vi "App - analyze RUS V6.vi"() -> ()   [LabVIEW 2018] (continued)
"timestamp"=timestamp(3493798379 s since 1904-01-01), "Magn Field(T)"=0.0}, {"temperature"=62.245, "lorentzian"={"A (VHz)"=0.0, "f (Hz)"=0.0, "G (Hz)"=0.0, "phi(rad)"=0.0, "Q"=0.0, "Norm  Ampl"=0.0, "bg (V)"=0.0+0.0i, "4corners"={"z (-pi/2)"=0.0+0.0i, "z(inf)"=0.0+0.0i, "z (pi/2)"=0.0+0.0i, "z center"=0.0+0.0i, "z(0)"=0.0+0.0i, "radius"=0.0}}, "timestamp(min)"=1177.3000000044703, "timestamp"=timestamp(3493798459 s since 1904-01-01), "Magn Field(T)"=0.0}, {"temperature"=62.184, "lorentzian"={"A (VHz)"=0.0, "f (Hz)"=0.0, "G (Hz)"=0.0, "phi(rad)"=0.0, "Q"=0.0, "Norm  Ampl"=0.0, "bg (V)"=0.0+0.0i, "4corners"={"z (-pi/2)"=0.0+0.0i, "z(inf)"=0.0+0.0i, "z (pi/2)"=0.0+0.0i, "z center"=0.0+0.0i, "z(0)"=0.0+0.0i, "radius"=0.0}}, "timestamp(min)"=1178.6166666671634, "timestamp"=timestamp(3493798538 s since 1904-01-01), "Magn Field(T)"=0.0}, {"temperature"=62.127, "lorentzian"={"A (VHz)"=0.0, "f (Hz)"=0.0, "G (Hz)"=0.0, "phi(rad)"=0.0, "Q"=0.0, "Norm  Ampl"=0.0, "bg (V)"=0.0+0.0i, "4corners"={"z (-pi/2)"=0.0+0.0i, "z(inf)"=0.0+0.0i, "z (pi/2)"=0.0+0.0i, "z center"=0.0+0.0i, "z(0)"=0.0+0.0i, "radius"=0.0}}, "timestamp(min)"=1179.933333337307, "timestamp"=timestamp(3493798617 s since 1904-01-01), "Magn Field(T)"=0.0}, {"temperature"=62.069, "lorentzian"={"A (VHz)"=0.0, "f (Hz)"=0.0, "G (Hz)"=0.0, "phi(rad)"=0.0, "Q"=0.0, "Norm  Ampl"=0.0, "bg (V)"=0.0+0.0i, "4corners"={"z (-pi/2)"=0.0+0.0i, "z(inf)"=0.0+0.0i, "z (pi/2)"=0.0+0.0i, "z center"=0.0+0.0i, "z(0)"=0.0+0.0i, "radius"=0.0}}, "timestamp(min)"=1181.2666666656733, "timestamp"=timestamp(3493798697 s since 1904-01-01), "Magn Field(T)"=0.0}, {"temperature"=62.01, "lorentzian"={"A (VHz)"=0.0, "f (Hz)"=0.0, "G (Hz)"=0.0, "phi(rad)"=0.0, "Q"=0.0, "Norm  Ampl"=0.0, "bg (V)"=0.0+0.0i, "4corners"={"z (-pi/2)"=0.0+0.0i, "z(inf)"=0.0+0.0i, "z (pi/2)"=0.0+0.0i, "z center"=0.0+0.0i, "z(0)"=0.0+0.0i, "radius"=0.0}}, "timestamp(min)"=1182.5833333358169, "timestamp"=timestamp(3493798776 s since 1904-01-01), "Magn Field(T)"=0.0}, {"temperature"=61.951, "lorentzian"={"A (VHz)"=0.0, "f (Hz)"=0.0, "G (Hz)"=0.0, "phi(rad)"=0.0, "Q"=0.0, "Norm  Ampl"=0.0, "bg (V)"=0.0+0.0i, "4corners"={"z (-pi/2)"=0.0+0.0i, "z(inf)"=0.0+0.0i, "z (pi/2)"=0.0+0.0i, "z center"=0.0+0.0i, "z(0)"=0.0+0.0i, "radius"=0.0}}, "timestamp(min)"=1183.8999999985099, "timestamp"=timestamp(3493798855 s since 1904-01-01), "Magn Field(T)"=0.0}, {"temperature"=61.895, "lorentzian"={"A (VHz)"=0.0, "f (Hz)"=0.0, "G (Hz)"=0.0, "phi(rad)"=0.0, "Q"=0.0, "Norm  Ampl"=0.0, "bg (V)"=0.0+0.0i, "4corners"={"z (-pi/2)"=0.0+0.0i, "z(inf)"=0.0+0.0i, "z (pi/2)"=0.0+0.0i, "z center"=0.0+0.0i, "z(0)"=0.0+0.0i, "radius"=0.0}}, "timestamp(min)"=1185.2333333343267, "timestamp"=timestamp(3493798935 s since 1904-01-01), "Magn Field(T)"=0.0}, {"temperature"=61.834, "lorentzian"={"A (VHz)"=0.0, "f (Hz)"=0.0, "G (Hz)"=0.0, "phi(rad)"=0.0, "Q"=0.0, "Norm  Ampl"=0.0, "bg (V)"=0.0+0.0i, "4corners"={"z (-pi/2)"=0.0+0.0i, "z(inf)"=0.0+0.0i, "z (pi/2)"=0.0+0.0i, "z center"=0.0+0.0i, "z(0)"=0.0+0.0i, "radius"=0.0}}, "timestamp(min)"=1186.5500000044703, "timestamp"=timestamp(3493799014 s since 1904-01-01), "Magn Field(T)"=0.0}, {"temperature"=61.775, "lorentzian"={"A (VHz)"=0.0, "f (Hz)"=0.0, "G (Hz)"=0.0, "phi(rad)"=0.0, "Q"=0.0, "Norm  Ampl"=0.0, "bg (V)"=0.0+0.0i, "4corners"={"z (-pi/2)"=0.0+0.0i, "z(inf)"=0.0+0.0i, "z (pi/2)"=0.0+0.0i, "z center"=0.0+0.0i, "z(0)"=0.0+0.0i, "radius"=0.0}}, "timestamp(min)"=1187.8833333328366, "timestamp"=timestamp(3493799094 s since 1904-01-01), "Magn Field(T)"=0.0}, {"temperature"=61.716, "lorentzian"={"A (VHz)"=0.0, "f (Hz)"=0.0, "G (Hz)"=0.0, "phi(rad)"=0.0, "Q"=0.0, "Norm  Ampl"=0.0, "bg (V)"=0.0+0.0i, "4corners"={"z (-pi/2)"=0.0+0.0i, "z(inf)"=0.0+0.0i, "z (pi/2)"=0.0+0.0i, "z center"=0.0+0.0i, "z(0)"=0.0+0.0i, "radius"=0.0}}, "timestamp(min)"=1189.2000000029802, "timestamp"=timestamp(3493799173 s since 1904-01-01), "Magn Field(T)"=0.0}, {"temperature"=61.656, "lorentzian"={"A (VHz)"=0.0, "f (Hz)"=0.0, "G (Hz)"=0.0, "phi(rad)"=0.0, "Q"=0.0, "Norm  Ampl"=0.0, "bg (V)"=0.0+0.0i, "4corners"={"z (-pi/2)"=0.0+0.0i, "z(inf)"=0.0+0.0i, "z (pi/2)"=0.0+0.0i, "z center"=0.0+0.0i, "z(0)"=0.0+0.0i, "radius"=0.0}}, "timestamp(min)"=1190.5166666656733, "timestamp"=timestamp(3493799252 s since 1904-01-01), "Magn Field(T)"=0.0}, {"temperature"=61.601, "lorentzian"={"A (VHz)"=0.0, "f (Hz)"=0.0, "G (Hz)"=0.0, "phi(rad)"=0.0, "Q"=0.0, "Norm  Ampl"=0.0, "bg (V)"=0.0+0.0i, "4corners"={"z (-pi/2)"=0.0+0.0i, "z(inf)"=0.0+0.0i, "z (pi/2)"=0.0+0.0i, "z center"=0.0+0.0i, "z(0)"=0.0+0.0i, "radius"=0.0}}, "timestamp(min)"=1191.8500000014901, "timestamp"=timestamp(3493799332 s since 1904-01-01), "Magn Field(T)"=0.0}, {"temperature"=61.541, "lorentzian"={"A (VHz)"=0.0, "f (Hz)"=0.0, "G (Hz)"=0.0, "phi(rad)"=0.0, "Q"=0.0, "Norm  Ampl"=0.0, "bg (V)"=0.0+0.0i, "4corners"={"z (-pi/2)"=0.0+0.0i, "z(inf)"=0.0+0.0i, "z (pi/2)"=0.0+0.0i, "z center"=0.0+0.0i, "z(0)"=0.0+0.0i, "radius"=0.0}}, "timestamp(min)"=1193.1666666641831, "timestamp"=timestamp(3493799411 s since 1904-01-01), "Magn Field(T)"=0.0}, {"temperature"=61.482, "lorentzian"={"A (VHz)"=0.0, "f (Hz)"=0.0, "G (Hz)"=0.0, "phi(rad)"=0.0, "Q"=0.0, "Norm  Ampl"=0.0, "bg (V)"=0.0+0.0i, "4corners"={"z (-pi/2)"=0.0+0.0i, "z(inf)"=0.0+0.0i, "z (pi/2)"=0.0+0.0i, "z center"=0.0+0.0i, "z(0)"=0.0+0.0i, "radius"=0.0}}, "timestamp(min)"=1194.5, "timestamp"=timestamp(3493799491 s since 1904-01-01), "Magn Field(T)"=0.0}, {"temperature"=61.424, "lorentzian"={"A (VHz)"=0.0, "f (Hz)"=0.0, "G (Hz)"=0.0, "phi(rad)"=0.0, "Q"=0.0, "Norm  Ampl"=0.0, "bg (V)"=0.0+0.0i, "4corners"={"z (-pi/2)"=0.0+0.0i, "z(inf)"=0.0+0.0i, "z (pi/2)"=0.0+0.0i, "z center"=0.0+0.0i, "z(0)"=0.0+0.0i, "radius"=0.0}}, "timestamp(min)"=1195.8166666701436, "timestamp"=timestamp(3493799570 s since 1904-01-01), "Magn Field(T)"=0.0}, {"temperature"=61.367, "lorentzian"={"A (VHz)"=0.0, "f (Hz)"=0.0, "G (Hz)"=0.0, "phi(rad)"=0.0, "Q"=0.0, "Norm  Ampl"=0.0, "bg (V)"=0.0+0.0i, "4corners"={"z (-pi/2)"=0.0+0.0i, "z(inf)"=0.0+0.0i, "z (pi/2)"=0.0+0.0i, "z center"=0.0+0.0i, "z(0)"=0.0+0.0i, "radius"=0.0}}, "timestamp(min)"=1197.1333333328366, "timestamp"=timestamp(3493799649 s since 1904-01-01), "Magn Field(T)"=0.0}, {"temperature"=61.307, "lorentzian"={"A (VHz)"=0.0, "f (Hz)"=0.0, "G (Hz)"=0.0, "phi(rad)"=0.0, "Q"=0.0, "Norm  Ampl"=0.0, "bg (V)"=0.0+0.0i, "4corners"={"z (-pi/2)"=0.0+0.0i, "z(inf)"=0.0+0.0i, "z (pi/2)"=0.0+0.0i, "z center"=0.0+0.0i, "z(0)"=0.0+0.0i, "radius"=0.0}}, "timestamp(min)"=1198.4666666686535, "timestamp"=timestamp(3493799729 s since 1904-01-01), "Magn Field(T)"=0.0}, {"temperature"=61.247, "lorentzian"={"A (VHz)"=0.0, "f (Hz)"=0.0, "G (Hz)"=0.0, "phi(rad)"=0.0, "Q"=0.0, "Norm  Ampl"=0.0, "bg (V)"=0.0+0.0i, "4corners"={"z (-pi/2)"=0.0+0.0i, "z(inf)"=0.0+0.0i, "z (pi/2)"=0.0+0.0i, "z center"=0.0+0.0i, "z(0)"=0.0+0.0i, "radius"=0.0}}, "timestamp(min)"=1199.7833333313465, "timestamp"=timestamp(3493799808 s since 1904-01-01), "Magn Field(T)"=0.0}, {"temperature"=61.191, "lorentzian"={"A (VHz)"=0.0, "f (Hz)"=0.0, "G (Hz)"=0.0, "phi(rad)"=0.0, "Q"=0.0, "Norm  Ampl"=0.0, "bg (V)"=0.0+0.0i, "4corners"={"z (-pi/2)"=0.0+0.0i, "z(inf)"=0.0+0.0i, "z (pi/2)"=0.0+0.0i, "z center"=0.0+0.0i, "z(0)"=0.0+0.0i, "radius"=0.0}}, "timestamp(min)"=1201.1000000014901, "timestamp"=timestamp(3493799887 s since 1904-01-01), "Magn Field(T)"=0.0}, {"temperature"=61.13, "lorentzian"={"A (VHz)"=0.0, "f (Hz)"=0.0, "G (Hz)"=0.0, "phi(rad)"=0.0, "Q"=0.0, "Norm  Ampl"=0.0, "bg (V)"=0.0+0.0i, "4corners"={"z (-pi/2)"=0.0+0.0i, "z(inf)"=0.0+0.0i, "z (pi/2)"=0.0+0.0i, "z center"=0.0+0.0i, "z(0)"=0.0+0.0i, "radius"=0.0}}, "timestamp(min)"=1202.433333337307, "timestamp"=timestamp(3493799967 s since 1904-01-01), "Magn Field(T)"=0.0}, {"temperature"=61.073, "lorentzian"={"A (VHz)"=0.0, "f (Hz)"=0.0, "G (Hz)"=0.0, "phi(rad)"=0.0, "Q"=0.0, "Norm  Ampl"=0.0, "bg (V)"=0.0+0.0i, "4corners"={"z (-pi/2)"=0.0+0.0i, "z(inf)"=0.0+0.0i, "z (pi/2)"=0.0+0.0i, "z center"=0.0+0.0i, "z(0)"=0.0+0.0i, "radius"=0.0}}, "timestamp(min)"=1203.75, "timestamp"=timestamp(3493800046 s since 1904-01-01), "Magn Field(T)"=0.0}, {"temperature"=61.013, "lorentzian"={"A (VHz)"=0.0, "f (Hz)"=0.0, "G (Hz)"=0.0, "phi(rad)"=0.0, "Q"=0.0, "Norm  Ampl"=0.0, "bg (V)"=0.0+0.0i, "4corners"={"z (-pi/2)"=0.0+0.0i, "z(inf)"=0.0+0.0i, "z (pi/2)"=0.0+0.0i, "z center"=0.0+0.0i, "z(0)"=0.0+0.0i, "radius"=0.0}}, "timestamp(min)"=1205.0833333358169, "timestamp"=timestamp(3493800126 s since 1904-01-01), "Magn Field(T)"=0.0}, {"temperature"=60.953, "lorentzian"={"A (VHz)"=0.0, "f (Hz)"=0.0, "G (Hz)"=0.0, "phi(rad)"=0.0, "Q"=0.0, "Norm  Ampl"=0.0, "bg (V)"=0.0+0.0i, "4corners"={"z (-pi/2)"=0.0+0.0i, "z(inf)"=0.0+0.0i, "z (pi/2)"=0.0+0.0i, "z center"=0.0+0.0i, "z(0)"=0.0+0.0i, "radius"=0.0}}, "timestamp(min)"=1206.3999999985099, "timestamp"=timestamp(3493800205 s since 1904-01-01), "Magn Field(T)"=0.0}, {"temperature"=60.896, "lorentzian"={"A (VHz)"=0.0, "f (Hz)"=0.0, "G (Hz)"=0.0, "phi(rad)"=0.0, "Q"=0.0, "Norm  Ampl"=0.0, "bg (V)"=0.0+0.0i, "4corners"={"z (-pi/2)"=0.0+0.0i, "z(inf)"=0.0+0.0i, "z (pi/2)"=0.0+0.0i, "z center"=0.0+0.0i, "z(0)"=0.0+0.0i, "radius"=0.0}}, "timestamp(min)"=1207.7166666686535, "timestamp"=timestamp(3493800284 s since 1904-01-01), "Magn Field(T)"=0.0}, {"temperature"=60.837, "lorentzian"={"A (VHz)"=0.0, "f (Hz)"=0.0, "G (Hz)"=0.0, "phi(rad)"=0.0, "Q"=0.0, "Norm  Ampl"=0.0, "bg (V)"=0.0+0.0i, "4corners"={"z (-pi/2)"=0.0+0.0i, "z(inf)"=0.0+0.0i, "z (pi/2)"=0.0+0.0i, "z center"=0.0+0.0i, "z(0)"=0.0+0.0i, "radius"=0.0}}, "timestamp(min)"=1209.0500000044703, "timestamp"=timestamp(3493800364 s since 1904-01-01), "Magn Field(T)"=0.0}, {"temperature"=60.781, "lorentzian"={"A (VHz)"=0.0, "f (Hz)"=0.0, "G (Hz)"=0.0, "phi(rad)"=0.0, "Q"=0.0, "Norm  Ampl"=0.0, "bg (V)"=0.0+0.0i, "4corners"={"z (-pi/2)"=0.0+0.0i, "z(inf)"=0.0+0.0i, "z (pi/2)"=0.0+0.0i, "z center"=0.0+0.0i, "z(0)"=0.0+0.0i, "radius"=0.0}}, "timestamp(min)"=1210.3666666671634, "timestamp"=timestamp(3493800443 s since 1904-01-01), "Magn Field(T)"=0.0}, {"temperature"=60.72, "lorentzian"={"A (VHz)"=0.0, "f (Hz)"=0.0, "G (Hz)"=0.0, "phi(rad)"=0.0, "Q"=0.0, "Norm  Ampl"=0.0, "bg (V)"=0.0+0.0i, "4corners"={"z (-pi/2)"=0.0+0.0i, "z(inf)"=0.0+0.0i, "z (pi/2)"=0.0+0.0i, "z center"=0.0+0.0i, "z(0)"=0.0+0.0i, "radius"=0.0}}, "timestamp(min)"=1211.683333337307, "timestamp"=timestamp(3493800522 s since 1904-01-01), "Magn Field(T)"=0.0}, {"temperature"=60.659, "lorentzian"={"A (VHz)"=0.0, "f (Hz)"=0.0, "G (Hz)"=0.0, "phi(rad)"=0.0, "Q"=0.0, "Norm  Ampl"=0.0, "bg (V)"=0.0+0.0i, "4corners"={"z (-pi/2)"=0.0+0.0i, "z(inf)"=0.0+0.0i, "z (pi/2)"=0.0+0.0i, "z center"=0.0+0.0i, "z(0)"=0.0+0.0i, "radius"=0.0}}, "timestamp(min)"=1213.0166666656733, "timestamp"=timestamp(3493800602 s since 1904-01-01), "Magn Field(T)"=0.0}, {"temperature"=60.601, "lorentzian"={"A (VHz)"=0.0, "f (Hz)"=0.0, "G (Hz)"=0.0, "phi(rad)"=0.0, "Q"=0.0, "Norm  Ampl"=0.0, "bg (V)"=0.0+0.0i, "4corners"={"z (-pi/2)"=0.0+0.0i, "z(inf)"=0.0+0.0i, "z (pi/2)"=0.0+0.0i, "z center"=0.0+0.0i, "z(0)"=0.0+0.0i, "radius"=0.0}}, "timestamp(min)"=1214.3333333358169, "timestamp"=timestamp(3493800681 s since 1904-01-01), "Magn Field(T)"=0.0}, {"temperature"=60.545, "lorentzian"={"A (VHz)"=0.0, "f (Hz)"=0.0, "G (Hz)"=0.0, "phi(rad)"=0.0, "Q"=0.0, "Norm  Ampl"=0.0, "bg (V)"=0.0+0.0i, "4corners"={"z (-pi/2)"=0.0+0.0i, "z(inf)"=0.0+0.0i, "z (pi/2)"=0.0+0.0i, "z center"=0.0+0.0i, "z(0)"=0.0+0.0i, "radius"=0.0}}, "timestamp(min)"=1215.6666666641831, "timestamp"=timestamp(3493800761 s since 1904-01-01), "Magn Field(T)"=0.0}, {"temperature"=60.486, "lorentzian"={"A (VHz)"=0.0, "f (Hz)"=0.0, "G (Hz)"=0.0, "phi(rad)"=0.0, "Q"=0.0, "Norm  Ampl"=0.0, "bg (V)"=0.0+0.0i, "4corners"={"z (-pi/2)"=0.0+0.0i, "z(inf)"=0.0+0.0i, "z (pi/2)"=0.0+0.0i, "z center"=0.0+0.0i, "z(0)"=0.0+0.0i, "radius"=0.0}}, "timestamp(min)"=1216.9833333343267, "timestamp"=timestamp(3493800840 s since 1904-01-01), "Magn Field(T)"=0.0}, {"temperature"=60.426, "lorentzian"={"A (VHz)"=0.0, "f (Hz)"=0.0, "G (Hz)"=0.0, "phi(rad)"=0.0, "Q"=0.0, "Norm  Ampl"=0.0, "bg (V)"=0.0+0.0i, "4corners"={"z (-pi/2)"=0.0+0.0i, "z(inf)"=0.0+0.0i, "z (pi/2)"=0.0+0.0i, "z center"=0.0+0.0i, "z(0)"=0.0+0.0i, "radius"=0.0}}, "timestamp(min)"=1218.3000000044703, "timestamp"=timestamp(3493800919 s since 1904-01-01), "Magn Field(T)"=0.0}, {"temperature"=60.367, "lorentzian"={"A (VHz)"=0.0, "f (Hz)"=0.0, "G (Hz)"=0.0, "phi(rad)"=0.0, "Q"=0.0, "Norm  Ampl"=0.0, "bg (V)"=0.0+0.0i, "4corners"={"z (-pi/2)"=0.0+0.0i, "z(inf)"=0.0+0.0i, "z (pi/2)"=0.0+0.0i, "z center"=0.0+0.0i, "z(0)"=0.0+0.0i, "radius"=0.0}}, "timestamp(min)"=1219.6333333328366, "timestamp"=timestamp(3493800999 s since 1904-01-01), "Magn Field(T)"=0.0}, {"temperature"=60.308, "lorentzian"={"A (VHz)"=0.0, "f (Hz)"=0.0, "G (Hz)"=0.0, "phi(rad)"=0.0, "Q"=0.0, "Norm  Ampl"=0.0, "bg (V)"=0.0+0.0i, "4corners"={"z (-pi/2)"=0.0+0.0i, "z(inf)"=0.0+0.0i, "z (pi/2)"=0.0+0.0i, "z center"=0.0+0.0i, "z(0)"=0.0+0.0i, "radius"=0.0}}, "timestamp(min)"=1220.9500000029802, "timestamp"=timestamp(3493801078 s since 1904-01-01), "Magn Field(T)"=0.0}, {"temperature"=60.248, "lorentzian"={"A (VHz)"=0.0, "f (Hz)"=0.0, "G (Hz)"=0.0, "phi(rad)"=0.0, "Q"=0.0, "Norm  Ampl"=0.0, "bg (V)"=0.0+0.0i, "4corners"={"z (-pi/2)"=0.0+0.0i, "z(inf)"=0.0+0.0i, "z (pi/2)"=0.0+0.0i, "z center"=0.0+0.0i, "z(0)"=0.0+0.0i, "radius"=0.0}}, "timestamp(min)"=1222.2833333313465, "timestamp"=timestamp(3493801158 s since 1904-01-01), "Magn Field(T)"=0.0}, {"temperature"=60.19, "lorentzian"={"A (VHz)"=0.0, "f (Hz)"=0.0, "G (Hz)"=0.0, "phi(rad)"=0.0, "Q"=0.0, "Norm  Ampl"=0.0, "bg (V)"=0.0+0.0i, "4corners"={"z (-pi/2)"=0.0+0.0i, "z(inf)"=0.0+0.0i, "z (pi/2)"=0.0+0.0i, "z center"=0.0+0.0i, "z(0)"=0.0+0.0i, "radius"=0.0}}, "timestamp(min)"=1223.6000000014901, "timestamp"=timestamp(3493801237 s since 1904-01-01), "Magn Field(T)"=0.0}, {"temperature"=60.133, "lorentzian"={"A (VHz)"=0.0, "f (Hz)"=0.0, "G (Hz)"=0.0, "phi(rad)"=0.0, "Q"=0.0, "Norm  Ampl"=0.0, "bg (V)"=0.0+0.0i, "4corners"={"z (-pi/2)"=0.0+0.0i, "z(inf)"=0.0+0.0i, "z (pi/2)"=0.0+0.0i, "z center"=0.0+0.0i, "z(0)"=0.0+0.0i, "radius"=0.0}}, "timestamp(min)"=1224.9166666641831, "timestamp"=timestamp(3493801316 s since 1904-01-01), "Magn Field(T)"=0.0}, {"temperature"=60.073, "lorentzian"={"A (VHz)"=0.0, "f (Hz)"=0.0, "G (Hz)"=0.0, "phi(rad)"=0.0, "Q"=0.0, "Norm  Ampl"=0.0, "bg (V)"=0.0+0.0i, "4corners"={"z (-pi/2)"=0.0+0.0i, "z(inf)"=0.0+0.0i, "z (pi/2)"=0.0+0.0i, "z center"=0.0+0.0i, "z(0)"=0.0+0.0i, "radius"=0.0}}, "timestamp(min)"=1226.25, "timestamp"=timestamp(3493801396 s since 1904-01-01), "Magn Field(T)"=0.0}, {"temperature"=60.013, "lorentzian"={"A (VHz)"=0.0, "f (Hz)"=0.0, "G (Hz)"=0.0, "phi(rad)"=0.0, "Q"=0.0, "Norm  Ampl"=0.0, "bg (V)"=0.0+0.0i, "4corners"={"z (-pi/2)"=0.0+0.0i, "z(inf)"=0.0+0.0i, "z (pi/2)"=0.0+0.0i, "z center"=0.0+0.0i, "z(0)"=0.0+0.0i, "radius"=0.0}}, "timestamp(min)"=1227.5666666701436, "timestamp"=timestamp(3493801475 s since 1904-01-01), "Magn Field(T)"=0.0}, {"temperature"=59.955, "lorentzian"={"A (VHz)"=0.0, "f (Hz)"=0.0, "G (Hz)"=0.0, "phi(rad)"=0.0, "Q"=0.0, "Norm  Ampl"=0.0, "bg (V)"=0.0+0.0i, "4corners"={"z (-pi/2)"=0.0+0.0i, "z(inf)"=0.0+0.0i, "z (pi/2)"=0.0+0.0i, "z center"=0.0+0.0i, "z(0)"=0.0+0.0i, "radius"=0.0}}, "timestamp(min)"=1228.8833333328366, "timestamp"=timestamp(3493801554 s since 1904-01-01), "Magn Field(T)"=0.0}, {"temperature"=59.894, "lorentzian"={"A (VHz)"=0.0, "f (Hz)"=0.0, "G (Hz)"=0.0, "phi(rad)"=0.0, "Q"=0.0, "Norm  Ampl"=0.0, "bg (V)"=0.0+0.0i, "4corners"={"z (-pi/2)"=0.0+0.0i, "z(inf)"=0.0+0.0i, "z (pi/2)"=0.0+0.0i, "z center"=0.0+0.0i, "z(0)"=0.0+0.0i, "radius"=0.0}}, "timestamp(min)"=1230.2166666686535, "timestamp"=timestamp(3493801634 s since 1904-01-01), "Magn Field(T)"=0.0}, {"temperature"=59.839, "lorentzian"={"A (VHz)"=0.0, "f (Hz)"=0.0, "G (Hz)"=0.0, "phi(rad)"=0.0, "Q"=0.0, "Norm  Ampl"=0.0, "bg (V)"=0.0+0.0i, "4corners"={"z (-pi/2)"=0.0+0.0i, "z(inf)"=0.0+0.0i, "z (pi/2)"=0.0+0.0i, "z center"=0.0+0.0i, "z(0)"=0.0+0.0i, "radius"=0.0}}, "timestamp(min)"=1231.5333333313465, "timestamp"=timestamp(3493801713 s since 1904-01-01), "Magn Field(T)"=0.0}, {"temperature"=59.776, "lorentzian"={"A (VHz)"=0.0, "f (Hz)"=0.0, "G (Hz)"=0.0, "phi(rad)"=0.0, "Q"=0.0, "Norm  Ampl"=0.0, "bg (V)"=0.0+0.0i, "4corners"={"z (-pi/2)"=0.0+0.0i, "z(inf)"=0.0+0.0i, "z (pi/2)"=0.0+0.0i, "z center"=0.0+0.0i, "z(0)"=0.0+0.0i, "radius"=0.0}}, "timestamp(min)"=1232.8666666671634, "timestamp"=timestamp(3493801793 s since 1904-01-01), "Magn Field(T)"=0.0}, {"temperature"=59.72, "lorentzian"={"A (VHz)"=0.0, "f (Hz)"=0.0, "G (Hz)"=0.0, "phi(rad)"=0.0, "Q"=0.0, "Norm  Ampl"=0.0, "bg (V)"=0.0+0.0i, "4corners"={"z (-pi/2)"=0.0+0.0i, "z(inf)"=0.0+0.0i, "z (pi/2)"=0.0+0.0i, "z center"=0.0+0.0i, "z(0)"=0.0+0.0i, "radius"=0.0}}, "timestamp(min)"=1234.183333337307, "timestamp"=timestamp(3493801872 s since 1904-01-01), "Magn Field(T)"=0.0}, {"temperature"=59.661, "lorentzian"={"A (VHz)"=0.0, "f (Hz)"=0.0, "G (Hz)"=0.0, "phi(rad)"=0.0, "Q"=0.0, "Norm  Ampl"=0.0, "bg (V)"=0.0+0.0i, "4corners"={"z (-pi/2)"=0.0+0.0i, "z(inf)"=0.0+0.0i, "z (pi/2)"=0.0+0.0i, "z center"=0.0+0.0i, "z(0)"=0.0+0.0i, "radius"=0.0}}, "timestamp(min)"=1235.5, "timestamp"=timestamp(3493801951 s since 1904-01-01), "Magn Field(T)"=0.0}, {"temperature"=59.598, "lorentzian"={"A (VHz)"=0.0, "f (Hz)"=0.0, "G (Hz)"=0.0, "phi(rad)"=0.0, "Q"=0.0, "Norm  Ampl"=0.0, "bg (V)"=0.0+0.0i, "4corners"={"z (-pi/2)"=0.0+0.0i, "z(inf)"=0.0+0.0i, "z (pi/2)"=0.0+0.0i, "z center"=0.0+0.0i, "z(0)"=0.0+0.0i, "radius"=0.0}}, "timestamp(min)"=1236.8333333358169, "timestamp"=timestamp(3493802031 s since 1904-01-01), "Magn Field(T)"=0.0}, {"temperature"=59.54, "lorentzian"={"A (VHz)"=0.0, "f (Hz)"=0.0, "G (Hz)"=0.0, "phi(rad)"=0.0, "Q"=0.0, "Norm  Ampl"=0.0, "bg (V)"=0.0+0.0i, "4corners"={"z (-pi/2)"=0.0+0.0i, "z(inf)"=0.0+0.0i, "z (pi/2)"=0.0+0.0i, "z center"=0.0+0.0i, "z(0)"=0.0+0.0i, "radius"=0.0}}, "timestamp(min)"=1238.1499999985099, "timestamp"=timestamp(3493802110 s since 1904-01-01), "Magn Field(T)"=0.0}, {"temperature"=59.481, "lorentzian"={"A (VHz)"=0.0, "f (Hz)"=0.0, "G (Hz)"=0.0, "phi(rad)"=0.0, "Q"=0.0, "Norm  Ampl"=0.0, "bg (V)"=0.0+0.0i, "4corners"={"z (-pi/2)"=0.0+0.0i, "z(inf)"=0.0+0.0i, "z (pi/2)"=0.0+0.0i, "z center"=0.0+0.0i, "z(0)"=0.0+0.0i, "radius"=0.0}}, "timestamp(min)"=1239.4833333343267, "timestamp"=timestamp(3493802190 s since 1904-01-01), "Magn Field(T)"=0.0}, {"temperature"=59.422, "lorentzian"={"A (VHz)"=0.0, "f (Hz)"=0.0, "G (Hz)"=0.0, "phi(rad)"=0.0, "Q"=0.0, "Norm  Ampl"=0.0, "bg (V)"=0.0+0.0i, "4corners"={"z (-pi/2)"=0.0+0.0i, "z(inf)"=0.0+0.0i, "z (pi/2)"=0.0+0.0i, "z center"=0.0+0.0i, "z(0)"=0.0+0.0i, "radius"=0.0}}, "timestamp(min)"=1240.8000000044703, "timestamp"=timestamp(3493802269 s since 1904-01-01), "Magn Field(T)"=0.0}, {"temperature"=59.365, "lorentzian"={"A (VHz)"=0.0, "f (Hz)"=0.0, "G (Hz)"=0.0, "phi(rad)"=0.0, "Q"=0.0, "Norm  Ampl"=0.0, "bg (V)"=0.0+0.0i, "4corners"={"z (-pi/2)"=0.0+0.0i, "z(inf)"=0.0+0.0i, "z (pi/2)"=0.0+0.0i, "z center"=0.0+0.0i, "z(0)"=0.0+0.0i, "radius"=0.0}}, "timestamp(min)"=1242.1166666671634, "timestamp"=timestamp(3493802348 s since 1904-01-01), "Magn Field(T)"=0.0}, {"temperature"=59.302, "lorentzian"={"A (VHz)"=0.0, "f (Hz)"=0.0, "G (Hz)"=0.0, "phi(rad)"=0.0, "Q"=0.0, "Norm  Ampl"=0.0, "bg (V)"=0.0+0.0i, "4corners"={"z (-pi/2)"=0.0+0.0i, "z(inf)"=0.0+0.0i, "z (pi/2)"=0.0+0.0i, "z center"=0.0+0.0i, "z(0)"=0.0+0.0i, "radius"=0.0}}, "timestamp(min)"=1243.4500000029802, "timestamp"=timestamp(3493802428 s since 1904-01-01), "Magn Field(T)"=0.0}, {"temperature"=59.243, "lorentzian"={"A (VHz)"=0.0, "f (Hz)"=0.0, "G (Hz)"=0.0, "phi(rad)"=0.0, "Q"=0.0, "Norm  Ampl"=0.0, "bg (V)"=0.0+0.0i, "4corners"={"z (-pi/2)"=0.0+0.0i, "z(inf)"=0.0+0.0i, "z (pi/2)"=0.0+0.0i, "z center"=0.0+0.0i, "z(0)"=0.0+0.0i, "radius"=0.0}}, "timestamp(min)"=1244.7666666656733, "timestamp"=timestamp(3493802507 s since 1904-01-01), "Magn Field(T)"=0.0}, {"temperature"=59.186, "lorentzian"={"A (VHz)"=0.0, "f (Hz)"=0.0, "G (Hz)"=0.0, "phi(rad)"=0.0, "Q"=0.0, "Norm  Ampl"=0.0, "bg (V)"=0.0+0.0i, "4corners"={"z (-pi/2)"=0.0+0.0i, "z(inf)"=0.0+0.0i, "z (pi/2)"=0.0+0.0i, "z center"=0.0+0.0i, "z(0)"=0.0+0.0i, "radius"=0.0}}, "timestamp(min)"=1246.0833333358169, "timestamp"=timestamp(3493802586 s since 1904-01-01), "Magn Field(T)"=0.0}, {"temperature"=59.124, "lorentzian"={"A (VHz)"=0.0, "f (Hz)"=0.0, "G (Hz)"=0.0, "phi(rad)"=0.0, "Q"=0.0, "Norm  Ampl"=0.0, "bg (V)"=0.0+0.0i, "4corners"={"z (-pi/2)"=0.0+0.0i, "z(inf)"=0.0+0.0i, "z (pi/2)"=0.0+0.0i, "z center"=0.0+0.0i, "z(0)"=0.0+0.0i, "radius"=0.0}}, "timestamp(min)"=1247.4166666641831, "timestamp"=timestamp(3493802666 s since 1904-01-01), "Magn Field(T)"=0.0}, {"temperature"=59.067, "lorentzian"={"A (VHz)"=0.0, "f (Hz)"=0.0, "G (Hz)"=0.0, "phi(rad)"=0.0, "Q"=0.0, "Norm  Ampl"=0.0, "bg (V)"=0.0+0.0i, "4corners"={"z (-pi/2)"=0.0+0.0i, "z(inf)"=0.0+0.0i, "z (pi/2)"=0.0+0.0i, "z center"=0.0+0.0i, "z(0)"=0.0+0.0i, "radius"=0.0}}, "timestamp(min)"=1248.7333333343267, "timestamp"=timestamp(3493802745 s since 1904-01-01), "Magn Field(T)"=0.0}, {"temperature"=59.005, "lorentzian"={"A (VHz)"=0.0, "f (Hz)"=0.0, "G (Hz)"=0.0, "phi(rad)"=0.0, "Q"=0.0, "Norm  Ampl"=0.0, "bg (V)"=0.0+0.0i, "4corners"={"z (-pi/2)"=0.0+0.0i, "z(inf)"=0.0+0.0i, "z (pi/2)"=0.0+0.0i, "z center"=0.0+0.0i, "z(0)"=0.0+0.0i, "radius"=0.0}}, "timestamp(min)"=1250.0666666701436, "timestamp"=timestamp(3493802825 s since 1904-01-01), "Magn Field(T)"=0.0}, {"temperature"=58.947, "lorentzian"={"A (VHz)"=0.0, "f (Hz)"=0.0, "G (Hz)"=0.0, "phi(rad)"=0.0, "Q"=0.0, "Norm  Ampl"=0.0, "bg (V)"=0.0+0.0i, "4corners"={"z (-pi/2)"=0.0+0.0i, "z(inf)"=0.0+0.0i, "z (pi/2)"=0.0+0.0i, "z center"=0.0+0.0i, "z(0)"=0.0+0.0i, "radius"=0.0}}, "timestamp(min)"=1251.3833333328366, "timestamp"=timestamp(3493802904 s since 1904-01-01), "Magn Field(T)"=0.0}, {"temperature"=58.886, "lorentzian"={"A (VHz)"=0.0, "f (Hz)"=0.0, "G (Hz)"=0.0, "phi(rad)"=0.0, "Q"=0.0, "Norm  Ampl"=0.0, "bg (V)"=0.0+0.0i, "4corners"={"z (-pi/2)"=0.0+0.0i, "z(inf)"=0.0+0.0i, "z (pi/2)"=0.0+0.0i, "z center"=0.0+0.0i, "z(0)"=0.0+0.0i, "radius"=0.0}}, "timestamp(min)"=1252.7000000029802, "timestamp"=timestamp(3493802983 s since 1904-01-01), "Magn Field(T)"=0.0}, {"temperature"=58.831, "lorentzian"={"A (VHz)"=0.0, "f (Hz)"=0.0, "G (Hz)"=0.0, "phi(rad)"=0.0, "Q"=0.0, "Norm  Ampl"=0.0, "bg (V)"=0.0+0.0i, "4corners"={"z (-pi/2)"=0.0+0.0i, "z(inf)"=0.0+0.0i, "z (pi/2)"=0.0+0.0i, "z center"=0.0+0.0i, "z(0)"=0.0+0.0i, "radius"=0.0}}, "timestamp(min)"=1254.0333333313465, "timestamp"=timestamp(3493803063 s since 1904-01-01), "Magn Field(T)"=0.0}, {"temperature"=58.769, "lorentzian"={"A (VHz)"=0.0, "f (Hz)"=0.0, "G (Hz)"=0.0, "phi(rad)"=0.0, "Q"=0.0, "Norm  Ampl"=0.0, "bg (V)"=0.0+0.0i, "4corners"={"z (-pi/2)"=0.0+0.0i, "z(inf)"=0.0+0.0i, "z (pi/2)"=0.0+0.0i, "z center"=0.0+0.0i, "z(0)"=0.0+0.0i, "radius"=0.0}}, "timestamp(min)"=1255.3500000014901, "timestamp"=timestamp(3493803142 s since 1904-01-01), "Magn Field(T)"=0.0}, {"temperature"=58.708, "lorentzian"={"A (VHz)"=0.0, "f (Hz)"=0.0, "G (Hz)"=0.0, "phi(rad)"=0.0, "Q"=0.0, "Norm  Ampl"=0.0, "bg (V)"=0.0+0.0i, "4corners"={"z (-pi/2)"=0.0+0.0i, "z(inf)"=0.0+0.0i, "z (pi/2)"=0.0+0.0i, "z center"=0.0+0.0i, "z(0)"=0.0+0.0i, "radius"=0.0}}, "timestamp(min)"=1256.6666666641831, "timestamp"=timestamp(3493803221 s since 1904-01-01), "Magn Field(T)"=0.0}, {"temperature"=58.65, "lorentzian"={"A (VHz)"=0.0, "f (Hz)"=0.0, "G (Hz)"=0.0, "phi(rad)"=0.0, "Q"=0.0, "Norm  Ampl"=0.0, "bg (V)"=0.0+0.0i, "4corners"={"z (-pi/2)"=0.0+0.0i, "z(inf)"=0.0+0.0i, "z (pi/2)"=0.0+0.0i, "z center"=0.0+0.0i, "z(0)"=0.0+0.0i, "radius"=0.0}}, "timestamp(min)"=1258.0, "timestamp"=timestamp(3493803301 s since 1904-01-01), "Magn Field(T)"=0.0}, {"temperature"=58.59, "lorentzian"={"A (VHz)"=0.0, "f (Hz)"=0.0, "G (Hz)"=0.0, "phi(rad)"=0.0, "Q"=0.0, "Norm  Ampl"=0.0, "bg (V)"=0.0+0.0i, "4corners"={"z (-pi/2)"=0.0+0.0i, "z(inf)"=0.0+0.0i, "z (pi/2)"=0.0+0.0i, "z center"=0.0+0.0i, "z(0)"=0.0+0.0i, "radius"=0.0}}, "timestamp(min)"=1259.3166666701436, "timestamp"=timestamp(3493803380 s since 1904-01-01), "Magn Field(T)"=0.0}, {"temperature"=58.53, "lorentzian"={"A (VHz)"=0.0, "f (Hz)"=0.0, "G (Hz)"=0.0, "phi(rad)"=0.0, "Q"=0.0, "Norm  Ampl"=0.0, "bg (V)"=0.0+0.0i, "4corners"={"z (-pi/2)"=0.0+0.0i, "z(inf)"=0.0+0.0i, "z (pi/2)"=0.0+0.0i, "z center"=0.0+0.0i, "z(0)"=0.0+0.0i, "radius"=0.0}}, "timestamp(min)"=1260.6499999985099, "timestamp"=timestamp(3493803460 s since 1904-01-01), "Magn Field(T)"=0.0}, {"temperature"=58.469, "lorentzian"={"A (VHz)"=0.0, "f (Hz)"=0.0, "G (Hz)"=0.0, "phi(rad)"=0.0, "Q"=0.0, "Norm  Ampl"=0.0, "bg (V)"=0.0+0.0i, "4corners"={"z (-pi/2)"=0.0+0.0i, "z(inf)"=0.0+0.0i, "z (pi/2)"=0.0+0.0i, "z center"=0.0+0.0i, "z(0)"=0.0+0.0i, "radius"=0.0}}, "timestamp(min)"=1261.9666666686535, "timestamp"=timestamp(3493803539 s since 1904-01-01), "Magn Field(T)"=0.0}, {"temperature"=58.41, "lorentzian"={"A (VHz)"=0.0, "f (Hz)"=0.0, "G (Hz)"=0.0, "phi(rad)"=0.0, "Q"=0.0, "Norm  Ampl"=0.0, "bg (V)"=0.0+0.0i, "4corners"={"z (-pi/2)"=0.0+0.0i, "z(inf)"=0.0+0.0i, "z (pi/2)"=0.0+0.0i, "z center"=0.0+0.0i, "z(0)"=0.0+0.0i, "radius"=0.0}}, "timestamp(min)"=1263.2833333313465, "timestamp"=timestamp(3493803618 s since 1904-01-01), "Magn Field(T)"=0.0}, {"temperature"=58.353, "lorentzian"={"A (VHz)"=0.0, "f (Hz)"=0.0, "G (Hz)"=0.0, "phi(rad)"=0.0, "Q"=0.0, "Norm  Ampl"=0.0, "bg (V)"=0.0+0.0i, "4corners"={"z (-pi/2)"=0.0+0.0i, "z(inf)"=0.0+0.0i, "z (pi/2)"=0.0+0.0i, "z center"=0.0+0.0i, "z(0)"=0.0+0.0i, "radius"=0.0}}, "timestamp(min)"=1264.6166666671634, "timestamp"=timestamp(3493803698 s since 1904-01-01), "Magn Field(T)"=0.0}, {"temperature"=58.289, "lorentzian"={"A (VHz)"=0.0, "f (Hz)"=0.0, "G (Hz)"=0.0, "phi(rad)"=0.0, "Q"=0.0, "Norm  Ampl"=0.0, "bg (V)"=0.0+0.0i, "4corners"={"z (-pi/2)"=0.0+0.0i, "z(inf)"=0.0+0.0i, "z (pi/2)"=0.0+0.0i, "z center"=0.0+0.0i, "z(0)"=0.0+0.0i, "radius"=0.0}}, "timestamp(min)"=1265.933333337307, "timestamp"=timestamp(3493803777 s since 1904-01-01), "Magn Field(T)"=0.0}, {"temperature"=58.232, "lorentzian"={"A (VHz)"=0.0, "f (Hz)"=0.0, "G (Hz)"=0.0, "phi(rad)"=0.0, "Q"=0.0, "Norm  Ampl"=0.0, "bg (V)"=0.0+0.0i, "4corners"={"z (-pi/2)"=0.0+0.0i, "z(inf)"=0.0+0.0i, "z (pi/2)"=0.0+0.0i, "z center"=0.0+0.0i, "z(0)"=0.0+0.0i, "radius"=0.0}}, "timestamp(min)"=1267.2666666656733, "timestamp"=timestamp(3493803857 s since 1904-01-01), "Magn Field(T)"=0.0}, {"temperature"=58.173, "lorentzian"={"A (VHz)"=0.0, "f (Hz)"=0.0, "G (Hz)"=0.0, "phi(rad)"=0.0, "Q"=0.0, "Norm  Ampl"=0.0, "bg (V)"=0.0+0.0i, "4corners"={"z (-pi/2)"=0.0+0.0i, "z(inf)"=0.0+0.0i, "z (pi/2)"=0.0+0.0i, "z center"=0.0+0.0i, "z(0)"=0.0+0.0i, "radius"=0.0}}, "timestamp(min)"=1268.5833333358169, "timestamp"=timestamp(3493803936 s since 1904-01-01), "Magn Field(T)"=0.0}, {"temperature"=58.111, "lorentzian"={"A (VHz)"=0.0, "f (Hz)"=0.0, "G (Hz)"=0.0, "phi(rad)"=0.0, "Q"=0.0, "Norm  Ampl"=0.0, "bg (V)"=0.0+0.0i, "4corners"={"z (-pi/2)"=0.0+0.0i, "z(inf)"=0.0+0.0i, "z (pi/2)"=0.0+0.0i, "z center"=0.0+0.0i, "z(0)"=0.0+0.0i, "radius"=0.0}}, "timestamp(min)"=1269.8999999985099, "timestamp"=timestamp(3493804015 s since 1904-01-01), "Magn Field(T)"=0.0}, {"temperature"=58.052, "lorentzian"={"A (VHz)"=0.0, "f (Hz)"=0.0, "G (Hz)"=0.0, "phi(rad)"=0.0, "Q"=0.0, "Norm  Ampl"=0.0, "bg (V)"=0.0+0.0i, "4corners"={"z (-pi/2)"=0.0+0.0i, "z(inf)"=0.0+0.0i, "z (pi/2)"=0.0+0.0i, "z center"=0.0+0.0i, "z(0)"=0.0+0.0i, "radius"=0.0}}, "timestamp(min)"=1271.2333333343267, "timestamp"=timestamp(3493804095 s since 1904-01-01), "Magn Field(T)"=0.0}, {"temperature"=57.991, "lorentzian"={"A (VHz)"=0.0, "f (Hz)"=0.0, "G (Hz)"=0.0, "phi(rad)"=0.0, "Q"=0.0, "Norm  Ampl"=0.0, "bg (V)"=0.0+0.0i, "4corners"={"z (-pi/2)"=0.0+0.0i, "z(inf)"=0.0+0.0i, "z (pi/2)"=0.0+0.0i, "z center"=0.0+0.0i, "z(0)"=0.0+0.0i, "radius"=0.0}}, "timestamp(min)"=1272.5500000044703, "timestamp"=timestamp(3493804174 s since 1904-01-01), "Magn Field(T)"=0.0}, {"temperature"=57.933, "lorentzian"={"A (VHz)"=0.0, "f (Hz)"=0.0, "G (Hz)"=0.0, "phi(rad)"=0.0, "Q"=0.0, "Norm  Ampl"=0.0, "bg (V)"=0.0+0.0i, "4corners"={"z (-pi/2)"=0.0+0.0i, "z(inf)"=0.0+0.0i, "z (pi/2)"=0.0+0.0i, "z center"=0.0+0.0i, "z(0)"=0.0+0.0i, "radius"=0.0}}, "timestamp(min)"=1273.8666666671634, "timestamp"=timestamp(3493804253 s since 1904-01-01), "Magn Field(T)"=0.0}, {"temperature"=57.871, "lorentzian"={"A (VHz)"=0.0, "f (Hz)"=0.0, "G (Hz)"=0.0, "phi(rad)"=0.0, "Q"=0.0, "Norm  Ampl"=0.0, "bg (V)"=0.0+0.0i, "4corners"={"z (-pi/2)"=0.0+0.0i, "z(inf)"=0.0+0.0i, "z (pi/2)"=0.0+0.0i, "z center"=0.0+0.0i, "z(0)"=0.0+0.0i, "radius"=0.0}}, "timestamp(min)"=1275.2000000029802, "timestamp"=timestamp(3493804333 s since 1904-01-01), "Magn Field(T)"=0.0}, {"temperature"=57.811, "lorentzian"={"A (VHz)"=0.0, "f (Hz)"=0.0, "G (Hz)"=0.0, "phi(rad)"=0.0, "Q"=0.0, "Norm  Ampl"=0.0, "bg (V)"=0.0+0.0i, "4corners"={"z (-pi/2)"=0.0+0.0i, "z(inf)"=0.0+0.0i, "z (pi/2)"=0.0+0.0i, "z center"=0.0+0.0i, "z(0)"=0.0+0.0i, "radius"=0.0}}, "timestamp(min)"=1276.5166666656733, "timestamp"=timestamp(3493804412 s since 1904-01-01), "Magn Field(T)"=0.0}, {"temperature"=57.752, "lorentzian"={"A (VHz)"=0.0, "f (Hz)"=0.0, "G (Hz)"=0.0, "phi(rad)"=0.0, "Q"=0.0, "Norm  Ampl"=0.0, "bg (V)"=0.0+0.0i, "4corners"={"z (-pi/2)"=0.0+0.0i, "z(inf)"=0.0+0.0i, "z (pi/2)"=0.0+0.0i, "z center"=0.0+0.0i, "z(0)"=0.0+0.0i, "radius"=0.0}}, "timestamp(min)"=1277.8500000014901, "timestamp"=timestamp(3493804492 s since 1904-01-01), "Magn Field(T)"=0.0}, {"temperature"=57.689, "lorentzian"={"A (VHz)"=0.0, "f (Hz)"=0.0, "G (Hz)"=0.0, "phi(rad)"=0.0, "Q"=0.0, "Norm  Ampl"=0.0, "bg (V)"=0.0+0.0i, "4corners"={"z (-pi/2)"=0.0+0.0i, "z(inf)"=0.0+0.0i, "z (pi/2)"=0.0+0.0i, "z center"=0.0+0.0i, "z(0)"=0.0+0.0i, "radius"=0.0}}, "timestamp(min)"=1279.1666666641831, "timestamp"=timestamp(3493804571 s since 1904-01-01), "Magn Field(T)"=0.0}, {"temperature"=57.629, "lorentzian"={"A (VHz)"=0.0, "f (Hz)"=0.0, "G (Hz)"=0.0, "phi(rad)"=0.0, "Q"=0.0, "Norm  Ampl"=0.0, "bg (V)"=0.0+0.0i, "4corners"={"z (-pi/2)"=0.0+0.0i, "z(inf)"=0.0+0.0i, "z (pi/2)"=0.0+0.0i, "z center"=0.0+0.0i, "z(0)"=0.0+0.0i, "radius"=0.0}}, "timestamp(min)"=1280.4833333343267, "timestamp"=timestamp(3493804650 s since 1904-01-01), "Magn Field(T)"=0.0}, {"temperature"=57.57, "lorentzian"={"A (VHz)"=0.0, "f (Hz)"=0.0, "G (Hz)"=0.0, "phi(rad)"=0.0, "Q"=0.0, "Norm  Ampl"=0.0, "bg (V)"=0.0+0.0i, "4corners"={"z (-pi/2)"=0.0+0.0i, "z(inf)"=0.0+0.0i, "z (pi/2)"=0.0+0.0i, "z center"=0.0+0.0i, "z(0)"=0.0+0.0i, "radius"=0.0}}, "timestamp(min)"=1281.8166666701436, "timestamp"=timestamp(3493804730 s since 1904-01-01), "Magn Field(T)"=0.0}, {"temperature"=57.51, "lorentzian"={"A (VHz)"=0.0, "f (Hz)"=0.0, "G (Hz)"=0.0, "phi(rad)"=0.0, "Q"=0.0, "Norm  Ampl"=0.0, "bg (V)"=0.0+0.0i, "4corners"={"z (-pi/2)"=0.0+0.0i, "z(inf)"=0.0+0.0i, "z (pi/2)"=0.0+0.0i, "z center"=0.0+0.0i, "z(0)"=0.0+0.0i, "radius"=0.0}}, "timestamp(min)"=1283.1333333328366, "timestamp"=timestamp(3493804809 s since 1904-01-01), "Magn Field(T)"=0.0}, {"temperature"=57.452, "lorentzian"={"A (VHz)"=0.0, "f (Hz)"=0.0, "G (Hz)"=0.0, "phi(rad)"=0.0, "Q"=0.0, "Norm  Ampl"=0.0, "bg (V)"=0.0+0.0i, "4corners"={"z (-pi/2)"=0.0+0.0i, "z(inf)"=0.0+0.0i, "z (pi/2)"=0.0+0.0i, "z center"=0.0+0.0i, "z(0)"=0.0+0.0i, "radius"=0.0}}, "timestamp(min)"=1284.4500000029802, "timestamp"=timestamp(3493804888 s since 1904-01-01), "Magn Field(T)"=0.0}, {"temperature"=57.391, "lorentzian"={"A (VHz)"=0.0, "f (Hz)"=0.0, "G (Hz)"=0.0, "phi(rad)"=0.0, "Q"=0.0, "Norm  Ampl"=0.0, "bg (V)"=0.0+0.0i, "4corners"={"z (-pi/2)"=0.0+0.0i, "z(inf)"=0.0+0.0i, "z (pi/2)"=0.0+0.0i, "z center"=0.0+0.0i, "z(0)"=0.0+0.0i, "radius"=0.0}}, "timestamp(min)"=1285.7833333313465, "timestamp"=timestamp(3493804968 s since 1904-01-01), "Magn Field(T)"=0.0}, {"temperature"=57.328, "lorentzian"={"A (VHz)"=0.0, "f (Hz)"=0.0, "G (Hz)"=0.0, "phi(rad)"=0.0, "Q"=0.0, "Norm  Ampl"=0.0, "bg (V)"=0.0+0.0i, "4corners"={"z (-pi/2)"=0.0+0.0i, "z(inf)"=0.0+0.0i, "z (pi/2)"=0.0+0.0i, "z center"=0.0+0.0i, "z(0)"=0.0+0.0i, "radius"=0.0}}, "timestamp(min)"=1287.1000000014901, "timestamp"=timestamp(3493805047 s since 1904-01-01), "Magn Field(T)"=0.0}, {"temperature"=57.27, "lorentzian"={"A (VHz)"=0.0, "f (Hz)"=0.0, "G (Hz)"=0.0, "phi(rad)"=0.0, "Q"=0.0, "Norm  Ampl"=0.0, "bg (V)"=0.0+0.0i, "4corners"={"z (-pi/2)"=0.0+0.0i, "z(inf)"=0.0+0.0i, "z (pi/2)"=0.0+0.0i, "z center"=0.0+0.0i, "z(0)"=0.0+0.0i, "radius"=0.0}}, "timestamp(min)"=1288.433333337307, "timestamp"=timestamp(3493805127 s since 1904-01-01), "Magn Field(T)"=0.0}, {"temperature"=57.209, "lorentzian"={"A (VHz)"=0.0, "f (Hz)"=0.0, "G (Hz)"=0.0, "phi(rad)"=0.0, "Q"=0.0, "Norm  Ampl"=0.0, "bg (V)"=0.0+0.0i, "4corners"={"z (-pi/2)"=0.0+0.0i, "z(inf)"=0.0+0.0i, "z (pi/2)"=0.0+0.0i, "z center"=0.0+0.0i, "z(0)"=0.0+0.0i, "radius"=0.0}}, "timestamp(min)"=1289.75, "timestamp"=timestamp(3493805206 s since 1904-01-01), "Magn Field(T)"=0.0}, {"temperature"=57.149, "lorentzian"={"A (VHz)"=0.0, "f (Hz)"=0.0, "G (Hz)"=0.0, "phi(rad)"=0.0, "Q"=0.0, "Norm  Ampl"=0.0, "bg (V)"=0.0+0.0i, "4corners"={"z (-pi/2)"=0.0+0.0i, "z(inf)"=0.0+0.0i, "z (pi/2)"=0.0+0.0i, "z center"=0.0+0.0i, "z(0)"=0.0+0.0i, "radius"=0.0}}, "timestamp(min)"=1291.0666666701436, "timestamp"=timestamp(3493805285 s since 1904-01-01), "Magn Field(T)"=0.0}, {"temperature"=57.087, "lorentzian"={"A (VHz)"=0.0, "f (Hz)"=0.0, "G (Hz)"=0.0, "phi(rad)"=0.0, "Q"=0.0, "Norm  Ampl"=0.0, "bg (V)"=0.0+0.0i, "4corners"={"z (-pi/2)"=0.0+0.0i, "z(inf)"=0.0+0.0i, "z (pi/2)"=0.0+0.0i, "z center"=0.0+0.0i, "z(0)"=0.0+0.0i, "radius"=0.0}}, "timestamp(min)"=1292.3999999985099, "timestamp"=timestamp(3493805365 s since 1904-01-01), "Magn Field(T)"=0.0}, {"temperature"=57.027, "lorentzian"={"A (VHz)"=0.0, "f (Hz)"=0.0, "G (Hz)"=0.0, "phi(rad)"=0.0, "Q"=0.0, "Norm  Ampl"=0.0, "bg (V)"=0.0+0.0i, "4corners"={"z (-pi/2)"=0.0+0.0i, "z(inf)"=0.0+0.0i, "z (pi/2)"=0.0+0.0i, "z center"=0.0+0.0i, "z(0)"=0.0+0.0i, "radius"=0.0}}, "timestamp(min)"=1293.7166666686535, "timestamp"=timestamp(3493805444 s since 1904-01-01), "Magn Field(T)"=0.0}, {"temperature"=56.968, "lorentzian"={"A (VHz)"=0.0, "f (Hz)"=0.0, "G (Hz)"=0.0, "phi(rad)"=0.0, "Q"=0.0, "Norm  Ampl"=0.0, "bg (V)"=0.0+0.0i, "4corners"={"z (-pi/2)"=0.0+0.0i, "z(inf)"=0.0+0.0i, "z (pi/2)"=0.0+0.0i, "z center"=0.0+0.0i, "z(0)"=0.0+0.0i, "radius"=0.0}}, "timestamp(min)"=1295.0500000044703, "timestamp"=timestamp(3493805524 s since 1904-01-01), "Magn Field(T)"=0.0}, {"temperature"=56.903, "lorentzian"={"A (VHz)"=0.0, "f (Hz)"=0.0, "G (Hz)"=0.0, "phi(rad)"=0.0, "Q"=0.0, "Norm  Ampl"=0.0, "bg (V)"=0.0+0.0i, "4corners"={"z (-pi/2)"=0.0+0.0i, "z(inf)"=0.0+0.0i, "z (pi/2)"=0.0+0.0i, "z center"=0.0+0.0i, "z(0)"=0.0+0.0i, "radius"=0.0}}, "timestamp(min)"=1296.3666666671634, "timestamp"=timestamp(3493805603 s since 1904-01-01), "Magn Field(T)"=0.0}, {"temperature"=56.847, "lorentzian"={"A (VHz)"=0.0, "f (Hz)"=0.0, "G (Hz)"=0.0, "phi(rad)"=0.0, "Q"=0.0, "Norm  Ampl"=0.0, "bg (V)"=0.0+0.0i, "4corners"={"z (-pi/2)"=0.0+0.0i, "z(inf)"=0.0+0.0i, "z (pi/2)"=0.0+0.0i, "z center"=0.0+0.0i, "z(0)"=0.0+0.0i, "radius"=0.0}}, "timestamp(min)"=1297.683333337307, "timestamp"=timestamp(3493805682 s since 1904-01-01), "Magn Field(T)"=0.0}, {"temperature"=56.789, "lorentzian"={"A (VHz)"=0.0, "f (Hz)"=0.0, "G (Hz)"=0.0, "phi(rad)"=0.0, "Q"=0.0, "Norm  Ampl"=0.0, "bg (V)"=0.0+0.0i, "4corners"={"z (-pi/2)"=0.0+0.0i, "z(inf)"=0.0+0.0i, "z (pi/2)"=0.0+0.0i, "z center"=0.0+0.0i, "z(0)"=0.0+0.0i, "radius"=0.0}}, "timestamp(min)"=1299.0166666656733, "timestamp"=timestamp(3493805762 s since 1904-01-01), "Magn Field(T)"=0.0}, {"temperature"=56.72, "lorentzian"={"A (VHz)"=0.0, "f (Hz)"=0.0, "G (Hz)"=0.0, "phi(rad)"=0.0, "Q"=0.0, "Norm  Ampl"=0.0, "bg (V)"=0.0+0.0i, "4corners"={"z (-pi/2)"=0.0+0.0i, "z(inf)"=0.0+0.0i, "z (pi/2)"=0.0+0.0i, "z center"=0.0+0.0i, "z(0)"=0.0+0.0i, "radius"=0.0}}, "timestamp(min)"=1300.3333333358169, "timestamp"=timestamp(3493805841 s since 1904-01-01), "Magn Field(T)"=0.0}, {"temperature"=56.664, "lorentzian"={"A (VHz)"=0.0, "f (Hz)"=0.0, "G (Hz)"=0.0, "phi(rad)"=0.0, "Q"=0.0, "Norm  Ampl"=0.0, "bg (V)"=0.0+0.0i, "4corners"={"z (-pi/2)"=0.0+0.0i, "z(inf)"=0.0+0.0i, "z (pi/2)"=0.0+0.0i, "z center"=0.0+0.0i, "z(0)"=0.0+0.0i, "radius"=0.0}}, "timestamp(min)"=1301.6499999985099, "timestamp"=timestamp(3493805920 s since 1904-01-01), "Magn Field(T)"=0.0}, {"temperature"=56.602, "lorentzian"={"A (VHz)"=0.0, "f (Hz)"=0.0, "G (Hz)"=0.0, "phi(rad)"=0.0, "Q"=0.0, "Norm  Ampl"=0.0, "bg (V)"=0.0+0.0i, "4corners"={"z (-pi/2)"=0.0+0.0i, "z(inf)"=0.0+0.0i, "z (pi/2)"=0.0+0.0i, "z center"=0.0+0.0i, "z(0)"=0.0+0.0i, "radius"=0.0}}, "timestamp(min)"=1302.9833333343267, "timestamp"=timestamp(3493806000 s since 1904-01-01), "Magn Field(T)"=0.0}, {"temperature"=56.543, "lorentzian"={"A (VHz)"=0.0, "f (Hz)"=0.0, "G (Hz)"=0.0, "phi(rad)"=0.0, "Q"=0.0, "Norm  Ampl"=0.0, "bg (V)"=0.0+0.0i, "4corners"={"z (-pi/2)"=0.0+0.0i, "z(inf)"=0.0+0.0i, "z (pi/2)"=0.0+0.0i, "z center"=0.0+0.0i, "z(0)"=0.0+0.0i, "radius"=0.0}}, "timestamp(min)"=1304.3000000044703, "timestamp"=timestamp(3493806079 s since 1904-01-01), "Magn Field(T)"=0.0}, {"temperature"=56.48, "lorentzian"={"A (VHz)"=0.0, "f (Hz)"=0.0, "G (Hz)"=0.0, "phi(rad)"=0.0, "Q"=0.0, "Norm  Ampl"=0.0, "bg (V)"=0.0+0.0i, "4corners"={"z (-pi/2)"=0.0+0.0i, "z(inf)"=0.0+0.0i, "z (pi/2)"=0.0+0.0i, "z center"=0.0+0.0i, "z(0)"=0.0+0.0i, "radius"=0.0}}, "timestamp(min)"=1305.6333333328366, "timestamp"=timestamp(3493806159 s since 1904-01-01), "Magn Field(T)"=0.0}, {"temperature"=56.419, "lorentzian"={"A (VHz)"=0.0, "f (Hz)"=0.0, "G (Hz)"=0.0, "phi(rad)"=0.0, "Q"=0.0, "Norm  Ampl"=0.0, "bg (V)"=0.0+0.0i, "4corners"={"z (-pi/2)"=0.0+0.0i, "z(inf)"=0.0+0.0i, "z (pi/2)"=0.0+0.0i, "z center"=0.0+0.0i, "z(0)"=0.0+0.0i, "radius"=0.0}}, "timestamp(min)"=1306.9500000029802, "timestamp"=timestamp(3493806238 s since 1904-01-01), "Magn Field(T)"=0.0}, {"temperature"=56.359, "lorentzian"={"A (VHz)"=0.0, "f (Hz)"=0.0, "G (Hz)"=0.0, "phi(rad)"=0.0, "Q"=0.0, "Norm  Ampl"=0.0, "bg (V)"=0.0+0.0i, "4corners"={"z (-pi/2)"=0.0+0.0i, "z(inf)"=0.0+0.0i, "z (pi/2)"=0.0+0.0i, "z center"=0.0+0.0i, "z(0)"=0.0+0.0i, "radius"=0.0}}, "timestamp(min)"=1308.2666666656733, "timestamp"=timestamp(3493806317 s since 1904-01-01), "Magn Field(T)"=0.0}, {"temperature"=56.297, "lorentzian"={"A (VHz)"=0.0, "f (Hz)"=0.0, "G (Hz)"=0.0, "phi(rad)"=0.0, "Q"=0.0, "Norm  Ampl"=0.0, "bg (V)"=0.0+0.0i, "4corners"={"z (-pi/2)"=0.0+0.0i, "z(inf)"=0.0+0.0i, "z (pi/2)"=0.0+0.0i, "z center"=0.0+0.0i, "z(0)"=0.0+0.0i, "radius"=0.0}}, "timestamp(min)"=1309.6000000014901, "timestamp"=timestamp(3493806397 s since 1904-01-01), "Magn Field(T)"=0.0}, {"temperature"=56.237, "lorentzian"={"A (VHz)"=0.0, "f (Hz)"=0.0, "G (Hz)"=0.0, "phi(rad)"=0.0, "Q"=0.0, "Norm  Ampl"=0.0, "bg (V)"=0.0+0.0i, "4corners"={"z (-pi/2)"=0.0+0.0i, "z(inf)"=0.0+0.0i, "z (pi/2)"=0.0+0.0i, "z center"=0.0+0.0i, "z(0)"=0.0+0.0i, "radius"=0.0}}, "timestamp(min)"=1310.9166666641831, "timestamp"=timestamp(3493806476 s since 1904-01-01), "Magn Field(T)"=0.0}, {"temperature"=56.174, "lorentzian"={"A (VHz)"=0.0, "f (Hz)"=0.0, "G (Hz)"=0.0, "phi(rad)"=0.0, "Q"=0.0, "Norm  Ampl"=0.0, "bg (V)"=0.0+0.0i, "4corners"={"z (-pi/2)"=0.0+0.0i, "z(inf)"=0.0+0.0i, "z (pi/2)"=0.0+0.0i, "z center"=0.0+0.0i, "z(0)"=0.0+0.0i, "radius"=0.0}}, "timestamp(min)"=1312.25, "timestamp"=timestamp(3493806556 s since 1904-01-01), "Magn Field(T)"=0.0}, {"temperature"=56.114, "lorentzian"={"A (VHz)"=0.0, "f (Hz)"=0.0, "G (Hz)"=0.0, "phi(rad)"=0.0, "Q"=0.0, "Norm  Ampl"=0.0, "bg (V)"=0.0+0.0i, "4corners"={"z (-pi/2)"=0.0+0.0i, "z(inf)"=0.0+0.0i, "z (pi/2)"=0.0+0.0i, "z center"=0.0+0.0i, "z(0)"=0.0+0.0i, "radius"=0.0}}, "timestamp(min)"=1313.5666666701436, "timestamp"=timestamp(3493806635 s since 1904-01-01), "Magn Field(T)"=0.0}, {"temperature"=56.051, "lorentzian"={"A (VHz)"=0.0, "f (Hz)"=0.0, "G (Hz)"=0.0, "phi(rad)"=0.0, "Q"=0.0, "Norm  Ampl"=0.0, "bg (V)"=0.0+0.0i, "4corners"={"z (-pi/2)"=0.0+0.0i, "z(inf)"=0.0+0.0i, 
